vi "Laurel TCP Initialize.vi"(6 "Connection Type":T1, 8 "Error In":errorcluster, 10 "Serial VISA":refnum<visa-resource-name>, 11 "Laurel IP Address":string) -> (0 "Error Out":errorcluster, 2 "Serial VISA Out":refnum<visa-resource-name>, 3 "Laurel Ref":refnum<k5>)   [LabVIEW 2019]
uses:
  Type Definitions/Laurel Connection Type.ctl
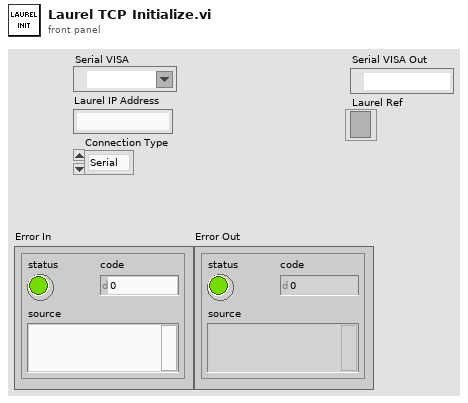
[diagram p1: front panel]
types:
  T1 = typedef "Laurel Connection Type.ctl" = enum16{"Serial", "TCP"}
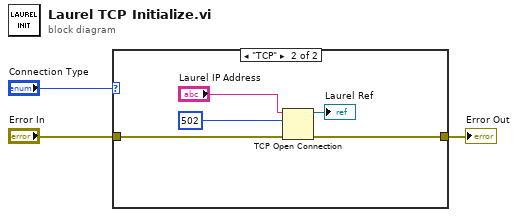
[diagram p0: block diagram]
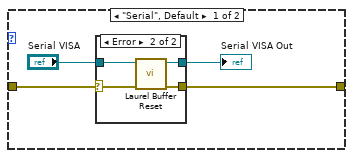
[diagram p2: hidden frame]
diagram:
  n1 = case shown="\"TCP\"" "Connection Type" {
    tunnel: [w6 w16] -> w3
    tunnel: "Error In" -> [w7 w15]
    frame "Serial", Default {
      n2 = case shown="Error" w7 {
        selector: w7 -> [w9 w11]
        tunnel: "Serial VISA" -> [w8 w10]
        tunnel: [w8 w13] -> w4
        tunnel: [w9 w12] -> w6
        frame No Error {
        }
        frame Error {
          n3 = call "Laurel Buffer Reset.vi"("error in (no error)"=w11, "VISA Refnum in"=w10) -> ("error out"=w12:errorcluster, "VISA Refnum out"=w13:refnum<visa-resource-name>)  [unwired: 8 in]
        }
      }
      "Serial VISA Out" <- w4
    }
    frame "TCP" {
      n4 = TCP Open Connection(address="Laurel IP Address", remote port or service name=u16 502, error in (no error)=w15) -> (connection ID=→"Laurel Ref":refnum<k5>, error out=w16:errorcluster)  [unwired: 2 in]
    }
  }
  "Error Out" <- w3
